vi "Query Multi Eval Meas List PERR DMRS Limit Check Results.vi"(7 "Window Position (Low)":i32(ring) items=["Low", "High"], 8 "error in (no error)":errorcluster, 9 "Result Type (Current)":i32(ring) items=["Current", "Average", "Extreme"], 10 "Instance (1)":T1=1, 11 "VISA resource name":refnum<visa-resource-name>) -> (0 "error out":errorcluster, 1 "PERR DRMS Limit Check Results":i32[](array[numeric]), 2 "Reliability":i32, 3 "VISA resource name out":refnum<visa-resource-name>)   [LabVIEW 2020, in "Rohde&Schwarz CMXP NR FR2 Measurement.lvlib"]
doc: "Returns the limit check results for the phase error DMRS values for low and high EVM window position, for all measured list mode segments.\n\nAttributes:\nRSCMXPNRFR2M_ATTR_QUERY_MULTI_EVAL_MEASUREMENT_LIST_PERR_DMRS_HIGH_AVERAGE_LIMIT_CHECK_RESULTS\nRSCMXPNRFR2M_ATTR_QUERY_MULTI_EVAL_MEASUREMENT_LIST_PERR_DMRS_HIGH_CURRENT_LIMIT_CHECK_RESULTS\nRSCMXPNRFR2M_ATTR_QUERY_MULTI_EVAL_MEASUREMENT_LIST_PERR_DMRS_HIGH_EXTREME_LIMIT_CHECK_RESULTS\nRSCMXPNRFR2M_ATTR_QUERY_MULTI_EVAL_MEASUREMENT_LIST_PERR_DMRS_LOW_AVERAGE_LIMIT_CHECK_RESULTS\nRSCMXPNRFR2M_ATTR_QUERY_MULTI_EVAL_MEASUREMENT_LIST_PERR_DMRS_LOW_CURRENT_LIMIT_CHECK_RESULTS\nRSCMXPNRFR2M_ATTR_QUERY_MULTI_EVAL_MEASUREMENT_LIST_PERR_DMRS_LOW_EXTREME_LIMIT_CHECK_RESULTS\n\nRemote-control commands:\nCALCulate:NRMMw:MEAS<i>:MEValuation:LIST:MODulation:PERRor:DMRS:HIGH:AVERage?\nCALCulate:NRMMw:MEAS<i>:MEValuation:LIST:MODulation:PERRor:DMRS:HIGH:CURRent?\nCALCulate:NRMMw:MEAS<i>:MEValuation:LIST:MODulation:PERRor:DMRS:HIGH:EXTReme?\nCALCulate:NRMMw:MEAS<i>:MEValuation:LIST:MODulation:PERRor:DMRS:LOW:AVERage?\nCALCulate:NRMMw:MEAS<i>:MEValuation:LIST:MODulation:PERRor:DMRS:LOW:CURRent?\nCALCulate:NRMMw:MEAS<i>:MEValuation:LIST:MODulation:PERRor:DMRS:LOW:EXTReme?"
uses:
  <instrlib>/Rohde&Schwarz CMXP NR FR2 Measurement/Rohde&Schwarz CMXP NR FR2 Measurement.lvlib
  <instrlib>/Rohde&Schwarz CMXP NR FR2 Measurement/Private/_Instance.ctl
  <instrlib>/Rohde&Schwarz CMXP NR FR2 Measurement/Private/rsidr_core.llb/rsidr_core.lvlib
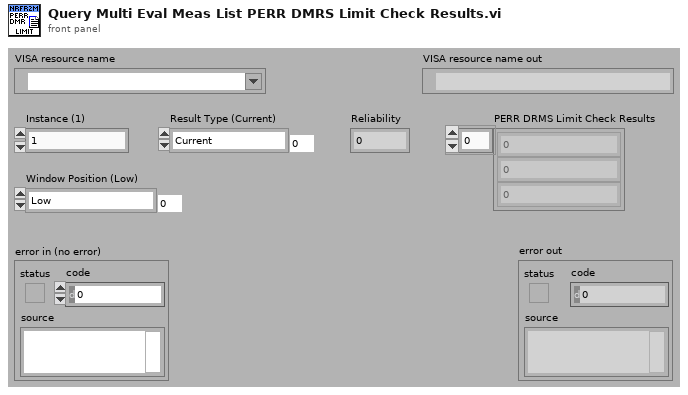
[diagram p1: front panel]
types:
  T1 = typedef "Rohde&Schwarz CMXP NR FR2 Measurement.lvlib/_Instance.ctl" = i32
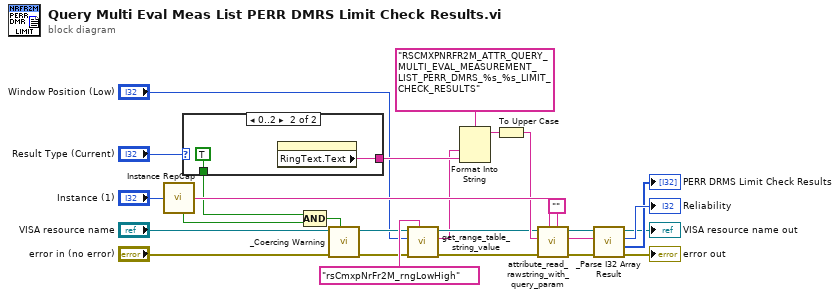
[diagram p0: block diagram]
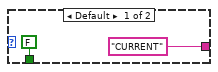
[diagram p2: hidden frame]
diagram:
  n1 = call <instrlib>:"Instance RepCap.vi"("Instance In"="Instance (1)") -> ("In Range?"=w23:bool, "RepCap Identifier Out"=w26:string)  [unwired: 1 in]
  n2 = case shown="0..2" "Result Type (Current)" {
    tunnel: ["CURRENT" w30] -> w24
    tunnel: [FALSE TRUE] -> w3
    frame Default {
    }
    frame 0..2 {
      n3 = property on="Result Type (Current)" class="Ring (strict)"() -> ("RingText.Text"=w30:string)  [unwired: 2 in, 2 out]
    }
  }
  n4 = Compound Arithmetic op=AND(w3, w23) -> (w22:bool)
  n5 = call <instrlib>:"_Coercing Warning.vi"("In Range?"=w22, "error in (no error)"="error in (no error)", "VISA resource name"="VISA resource name") -> ("error out"=w7:errorcluster, "VISA resource name out"=w8:refnum<visa-resource-name>)  [unwired: 7 in]
  n6 = call <instrlib>:"get_range_table_string_value.vi"("Range Table ID in"="rsCmxpNrFr2M_rngLowHigh", "error in"=w7, "I32 input"="Window Position (Low)", "VISA resource name"=w8) -> ("error out"=w5:errorcluster, "String Value out"=w1:string, "VISA resource name out"=w4:refnum<visa-resource-name>)  [unwired: 5 in]
  n7 = Format Into String(format string="RSCMXPNRFR2M_ATTR_QUERY_MULTI_EVAL_MEASUREMENT_LIST_PERR_DMRS_%s_%s_LIMIT_CHECK_RESULTS", w1, w24) -> (resulting string=w25:string)  [unwired: 2 in, 1 out]
  n8 = To Upper Case(1:w25) -> (0:w17:string)
  n9 = call <instrlib>:"attribute_read_rawstring_with_query_param.vi"("Query Parameter (None)"="" ("Empty String Constant"), "Repeated Capability"=w26, "error in"=w5, "Attribute ID"=w17, "VISA resource name"=w4) -> ("error out"=w20:errorcluster, "Raw String out"=w19:string, "VISA resource name out"=w18:refnum<visa-resource-name>)  [unwired: 4 in]
  n10 = call <instrlib>:"_Parse I32 Array Result.vi"("error in (no error)"=w20, "Input String"=w19, "VISA resource name"=w18) -> ("error out"=→"error out":errorcluster, "Results"=→"PERR DRMS Limit Check Results":i32[], "Reliability"=→"Reliability":i32, "VISA resource name out"=→"VISA resource name out":refnum<visa-resource-name>)  [unwired: 5 in]
